vi "ClosePCCamera.vi"(2 "error in (no error)":errorcluster, 3 "Camera Reference":i64) -> (0 "error out":errorcluster)   [LabVIEW 2022 SP3]
uses:
  <vilib>/addons/RoboLab/ImageProcessing/WindowsDriver/LVDS.dll
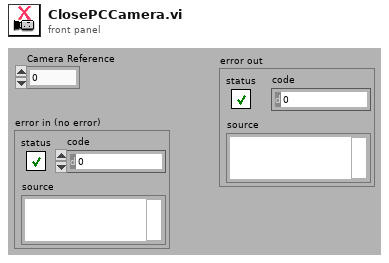
[diagram p1: front panel]
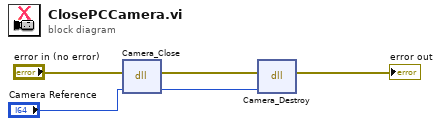
[diagram p0: block diagram]
diagram:
  n1 = dll-call lib="C:/Program Files (x86)/National Instruments/LabVIEW 2022/vi.lib/addons/RoboLab/ImageProcessing/WindowsDriver/LVDS.dll" fn="Camera_Close"(error in="error in (no error)", "cameraReference"="Camera Reference") -> (error out=w2:errorcluster, "cameraReference"=w1:i64)  [unwired: 3 in, 1 out]
  n2 = dll-call lib="C:/Program Files (x86)/National Instruments/LabVIEW 2022/vi.lib/addons/RoboLab/ImageProcessing/WindowsDriver/LVDS.dll" fn="Camera_Destroy"(error in=w2, "index"=w1) -> (error out=→"error out":errorcluster)  [unwired: 4 in, 1 out]
